vi "write_signals.vi"(8 "error in (no error)":errorcluster, 11 "DL090202ScanHead in":refnum<class "ScanHeadDL090202.lvclass">) -> (0 "error out":errorcluster, 2 "finished?":bool, 3 "DL090202ScanHead out":refnum<class "ScanHeadDL090202.lvclass">)   [LabVIEW 2010, in "ScanHeadDL090202.lvclass"]
uses:
  ScanHeadDL090202.lvclass
  SignalWriter/GenericSignalWriter/GenericSignalWriter/GenericSignalWriter.lvclass
  common/classes/ErrorController/ErrorController/class_data.vi
  common/classes/ErrorController/ErrorController/ErrorController.lvclass
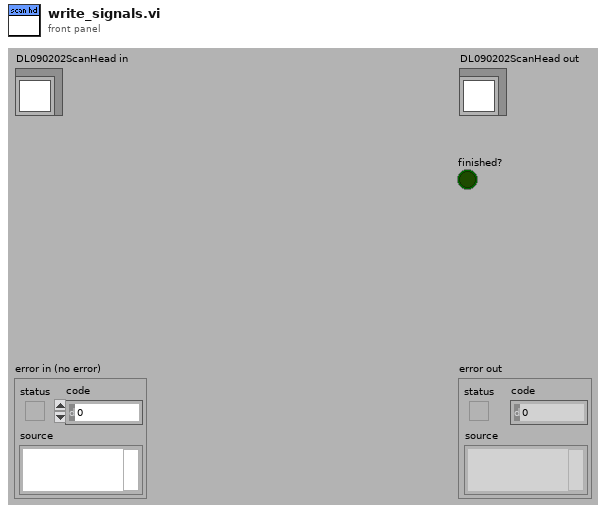
[diagram p1: front panel]
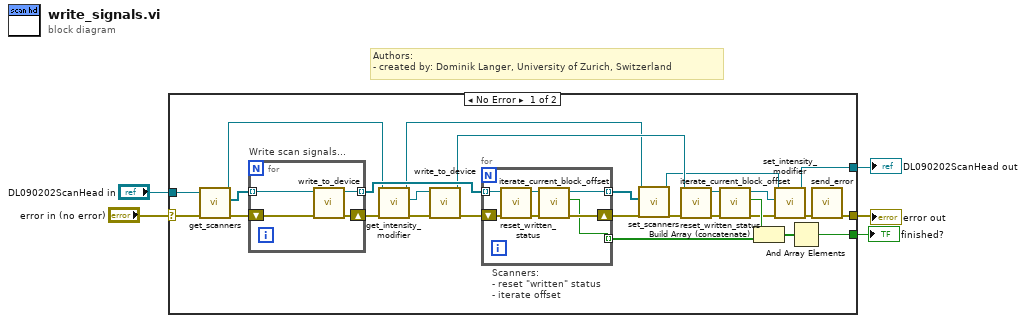
[diagram p0: block diagram]
diagram:
  # "Authors: \n- created by: Dominik Langer, University of Zurich, Switzerland"
  n1 = case shown="No Error" "error in (no error)" {
    selector: "error in (no error)" -> [w25 w45]
    tunnel: [w6 w45] -> w1
    tunnel: [w14 w44] -> w3
    tunnel: "DL090202ScanHead in" -> [w22 w44]
    tunnel: [w28 _] -> w2
    frame No Error {
      n2 = call-dynamic "get_scanners.vi"("error in (no error)"=w25, "DL090202ScanHead.lvclass in"=w22) -> ("error out"=w24:errorcluster, "scanners"=w23:refnum<class "GenericSignalWriter.lvclass">[], "DL090202ScanHead.lvclass out"=w9:refnum<class "ScanHeadDL090202.lvclass">)  [unwired: 7 in]
      n3 = for "Write scan signals..." {
        tunnel: w23 -> [w41] mode=indexing
        tunnel: [w43] -> w32 mode=indexing
        shift-right: [w40] -> w21
        shift-left: w24 -> [w42]
        n4 = call-dynamic "write_to_device.vi"("error in (no error)"=w42, "GenericWriteSignals in"=w41) -> ("error out"=w40:errorcluster, "GenericWriteSignals out"=w43:refnum<class "GenericSignalWriter.lvclass">)  [unwired: 1 in, 7 out]
      }
      n5 = call-dynamic "get_intensity_modifier.vi"("error in (no error)"=w21, "DL090202ScanHead.lvclass in"=w9) -> ("error out"=w20:errorcluster, "write signals"=w19:refnum<class "GenericSignalWriter.lvclass">, "DL090202ScanHead.lvclass out"=w8:refnum<class "ScanHeadDL090202.lvclass">)  [unwired: 7 in]
      n6 = call-dynamic "write_to_device.vi"("error in (no error)"=w20, "GenericWriteSignals in"=w19) -> ("error out"=w31:errorcluster, "GenericWriteSignals out"=w30:refnum<class "GenericSignalWriter.lvclass">)  [unwired: 1 in, 7 out]
      n7 = for "Scanners: \n- reset \"written\" status\n- iterate offset" {
        tunnel: w32 -> [w38] mode=indexing
        shift-right: [w35] -> w12
        shift-left: w31 -> [w39]
        tunnel: [w34] -> w13 mode=indexing
        tunnel: [w33] -> w26 mode=indexing
        n8 = call-dynamic "reset_written_status.vi"("error in (no error)"=w39, "GenericWriteSignals in"=w38) -> ("error out"=w37:errorcluster, "GenericWriteSignals out"=w36:refnum<class "GenericSignalWriter.lvclass">)  [unwired: 8 out]
        n9 = call-dynamic "iterate_current_block_offset.vi"("error in (no error)"=w37, "GenericWriteSignals in"=w36) -> ("error out"=w35:errorcluster, "finished?"=w33:bool, "GenericWriteSignals out"=w34:refnum<class "GenericSignalWriter.lvclass">)  [unwired: 7 out]
      }
      n10 = call-dynamic "set_scanners.vi"("error in (no error)"=w12, "scanners"=w13, "DL090202ScanHead.lvclass in"=w8) -> ("error out"=w11:errorcluster, "DL090202ScanHead.lvclass out"=w10:refnum<class "ScanHeadDL090202.lvclass">)  [unwired: 7 in]
      n11 = call-dynamic "reset_written_status.vi"("error in (no error)"=w11, "GenericWriteSignals in"=w30) -> ("error out"=w18:errorcluster, "GenericWriteSignals out"=w17:refnum<class "GenericSignalWriter.lvclass">)  [unwired: 8 out]
      n12 = call-dynamic "iterate_current_block_offset.vi"("error in (no error)"=w18, "GenericWriteSignals in"=w17) -> ("error out"=w15:errorcluster, "finished?"=w27:bool, "GenericWriteSignals out"=w16:refnum<class "GenericSignalWriter.lvclass">)  [unwired: 7 out]
      n13 = Build Array (concatenate)(w27, w26) -> (w29:bool[])
      n14 = call-dynamic "set_intensity_modifier.vi"("error in (no error)"=w15, "write signals"=w16, "DL090202ScanHead.lvclass in"=w10) -> ("error out"=w7:errorcluster, "DL090202ScanHead.lvclass out"=w14:refnum<class "ScanHeadDL090202.lvclass">)  [unwired: 7 in]
      n15 = And Array Elements(Boolean array=w29) -> (logical AND=w28:bool)
      n16 = call "send_error.vi"("error in (no error)"=w7) -> ("error out"=w6:errorcluster)  [unwired: 10 in]
    }
    frame Error {
    }
  }
  "error out" <- w1
  "DL090202ScanHead out" <- w3
  "finished?" <- w2
